vi "Phase III Globals.vi"() -> ()   [LabVIEW 2022 SP3]
uses:
  Controls/NS Data type.ctl
panel:
  in  "Reader url":refnum<k21>
  out "Connected?":bool
  in  "writer url":refnum<k21>
  out "Exit":bool
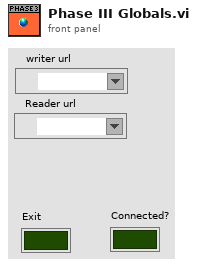
[diagram p1: front panel]
diagram:
